vi "ClassNameCacheWrite.vi"(10 "Class (child,parent)":T1[](array[typedef]), 11 "Map":T2) -> (3 "Map":T2)   [LabVIEW 2020, in "BlueSerialization.lvlib" / "BlueSerializer.lvclass"]
uses:
  BlueSerializer.lvclass
  ClassNameCacheMap.ctl
  ClassNameObj.ctl
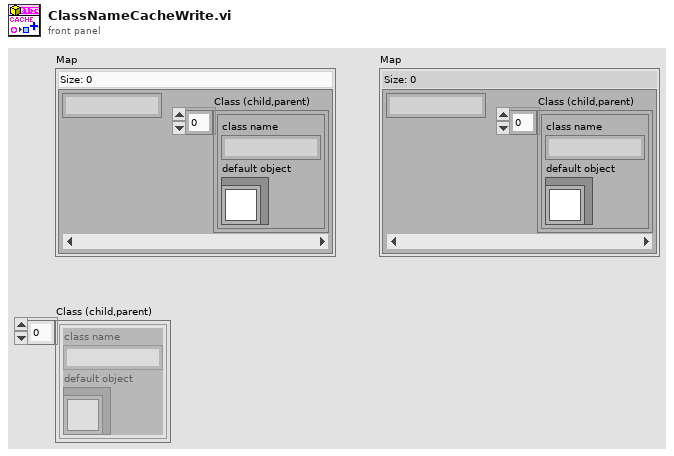
[diagram p1: front panel]
types:
  T1 = typedef "BlueSerialization.lvlib/BlueSerializer.lvclass/ClassNameObj.ctl" = cluster{"class name":string, "default object":refnum<class>}
  T2 = typedef "BlueSerialization.lvlib/BlueSerializer.lvclass/ClassNameCacheMap.ctl" = map{string, T1[]}
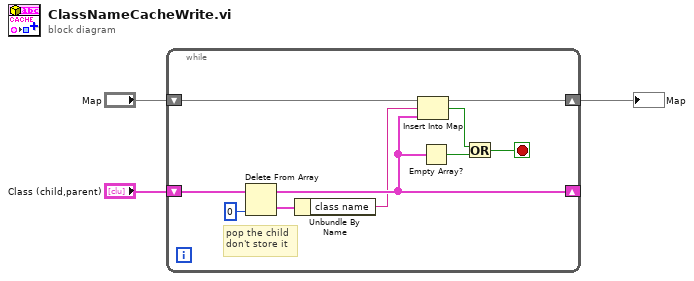
[diagram p0: block diagram]
diagram:
  n1 = while {
    shift-right: [w12] -> w2
    shift-left: "Map" -> [w13]
    shift-right: [w9] -> _
    shift-left: "Class (child,parent)" -> [w11]
    stop <- w6 stop-if-true
    # "pop the child\ndon't store it"
    n2 = Delete From Array(array=w11, index=0) -> (deleted portion=w5:T1, array with subset deleted=w9:T1[])  [unwired: 1 in]
    n3 = Unbundle By Name(w5) -> ("class name"=w4:string)
    n4 = Insert Into Map(map in=w13, key=w4, value=w9) -> (map out=w12:T2, key already included?=w7:bool)  [unwired: 1 out]
    n5 = Empty Array?(array=w9) -> (empty?=w8:bool)
    n6 = Or(x=w7, y=w8) -> (x .or. y?=w6:bool)
  }
  "Map" <- w2
